vi "dds_rom_mixer_filter_spi.vi"() -> ()   [LabVIEW 2018]
uses:
  <vilib>/Analysis/NI_AALBase.lvlib
panel:
  out "IVAL":i16
  in  "Load":bool
  in  "ADC Offset":u16
  in  "PID":cluster{"S":i16, "O":i16, "P":i16, "I":i8}
  in  "Port":refnum<visa-resource-name>="COM3"
  in  "Init":bool
  in  "DDS":T1(array[cluster])=[{"Frequency"=0, "Attenuation"=0, "Phase"=0.0}, {"Frequency"=0, "Attenuation"=0, "Phase"=0.0}] {"Phase" min=0.0 max=2.0 format="%.3f"; "Attenuation" max=15}
  in  "Y":u16(ring)=4 items=["DDS0", "DDS1", "ROM", "MIXER", "FILTER", "ADC0", "ADC1", "ADC2", "ADC12", "PID"]
  in  "X":u16(ring) items=["DDS0", "DDS1", "ROM", "MIXER", "FILTER", "ADC0", "ADC1", "ADC2", "ADC12", "PID"]
  in  "t":u16(ring) items=["DDS", "ROM", "MIXER", "FILTER", "DAC", "ADC", "PID"]
  in  "State":u16(ring) items=["IDLE", "TEST", "DDS_DAC", "DDS_DAC_FILTER", "ADC", "DDS_DAC_ADC", "DDS_DAC_ADC_MIXER_FILTER", "DDS_DAC_ADC_MIXER_FILTER_PID"]
  in  "Filter Param":u16=9 max=15
  in  "stop":bool
  out "Waveform Graph":i16[][](graph)
  out "XY Graph":cluster{i16[], i16[]}(graph)
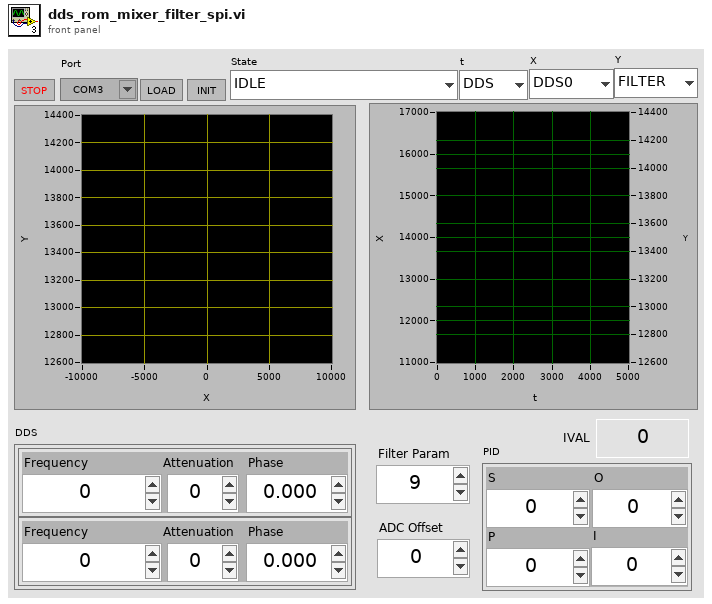
[diagram p1: front panel]
types:
  T1 = cluster{"Frequency":u16, "Attenuation":u16, "Phase":dbl}[]
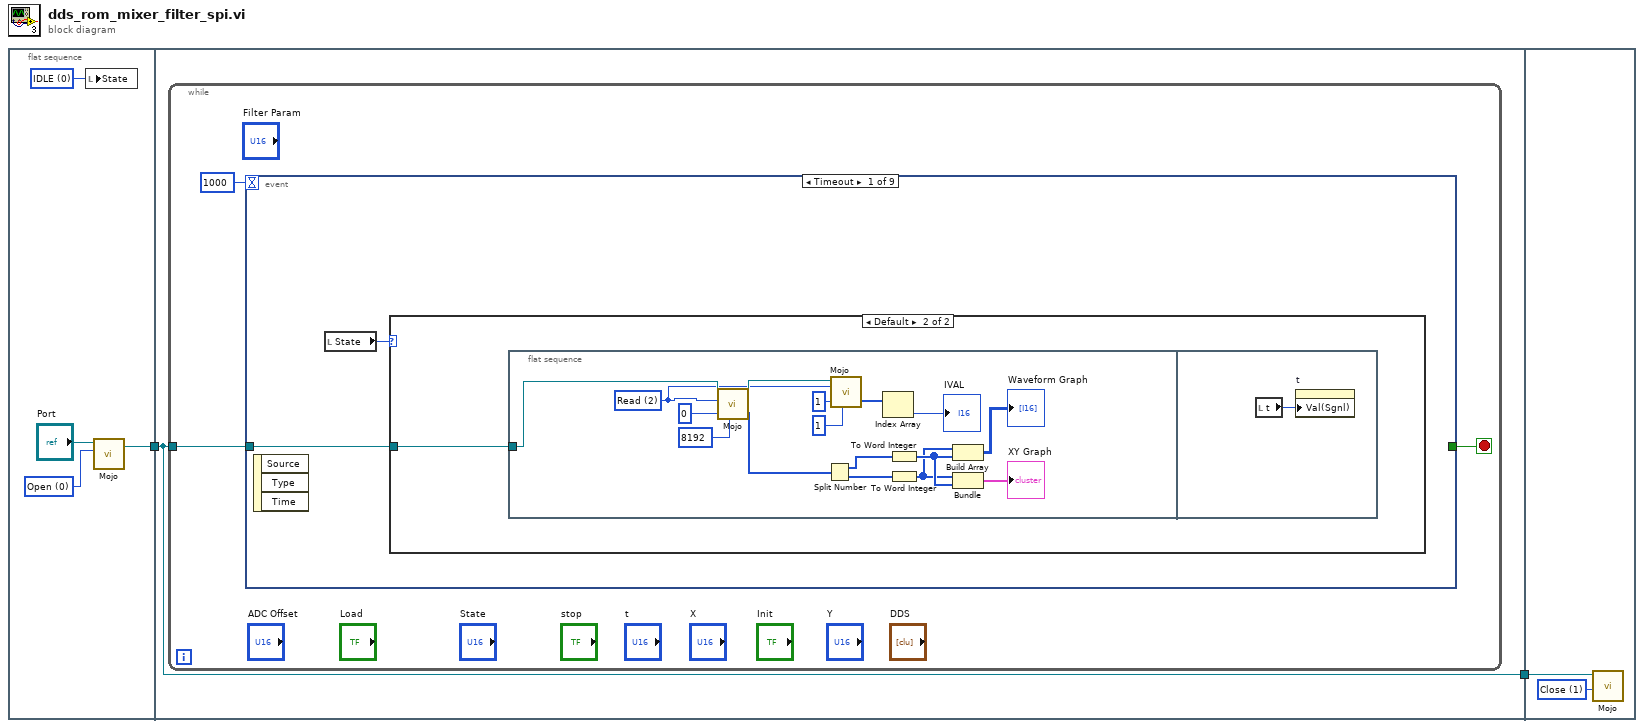
[diagram p0: block diagram]
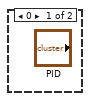
[diagram p2: hidden frame]
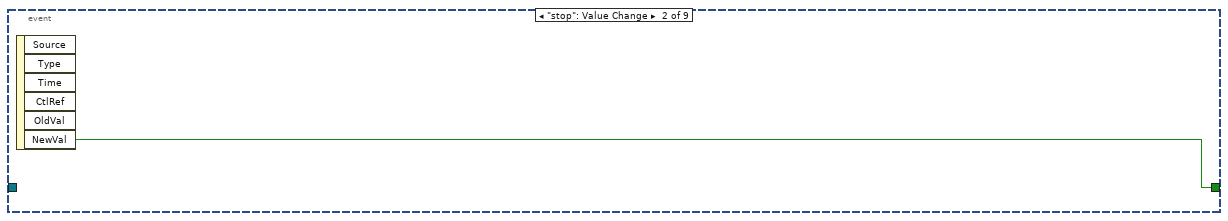
[diagram p3: hidden frame]
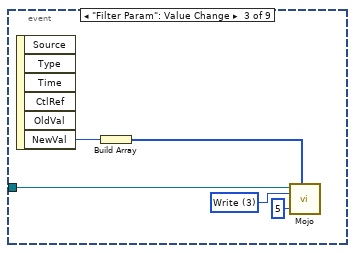
[diagram p4: hidden frame]
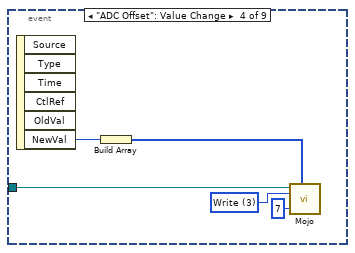
[diagram p5: hidden frame]
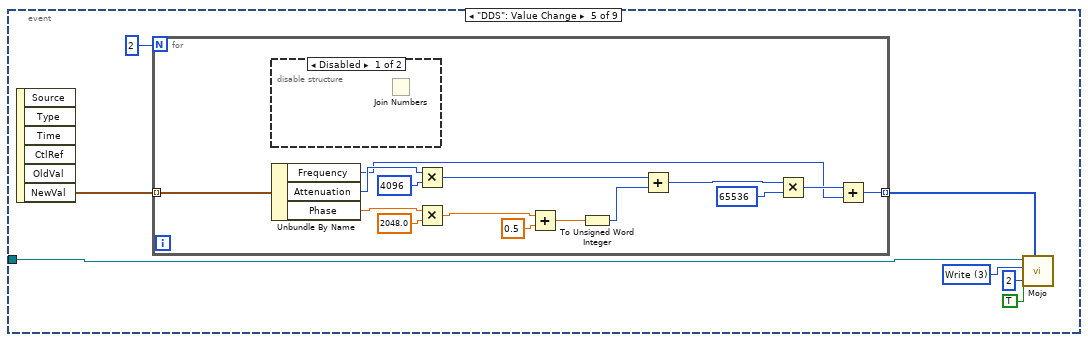
[diagram p6: hidden frame]
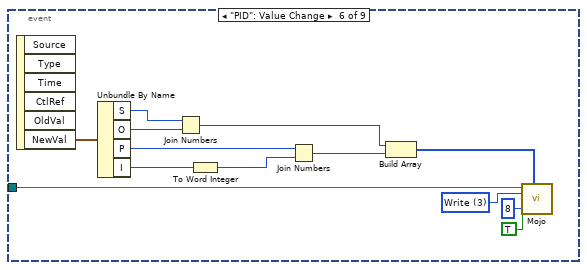
[diagram p8: hidden frame]
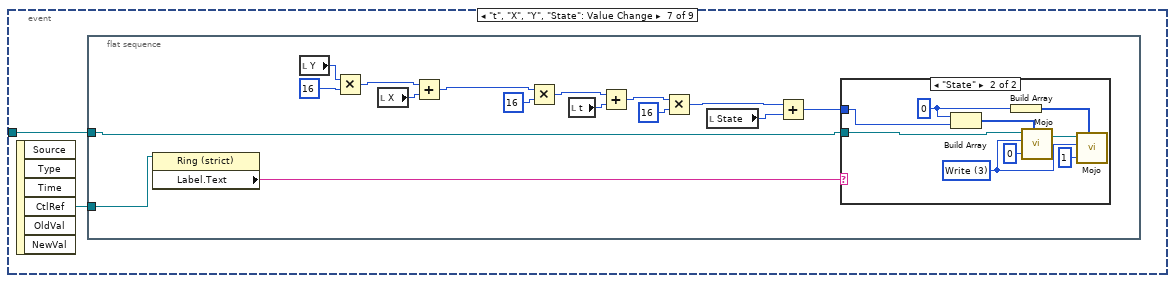
[diagram p9: hidden frame]
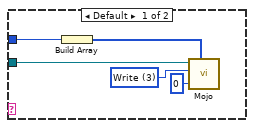
[diagram p10: hidden frame]
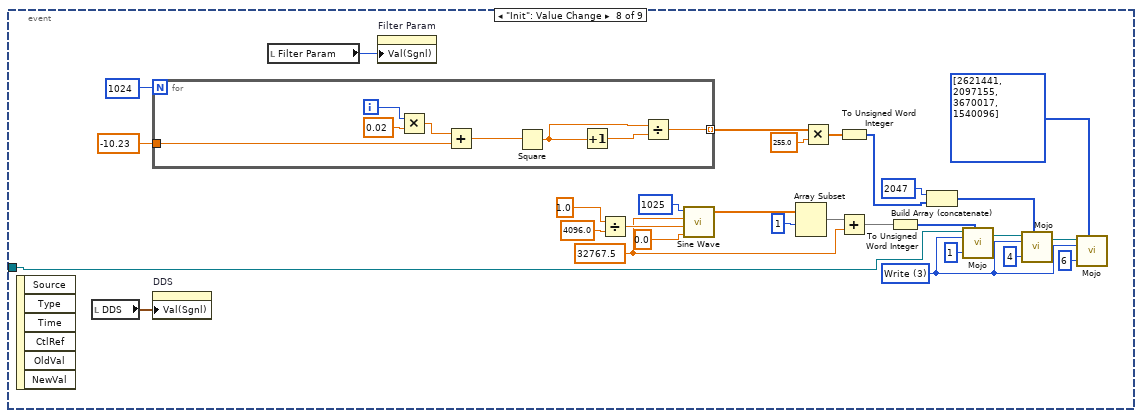
[diagram p11: hidden frame]
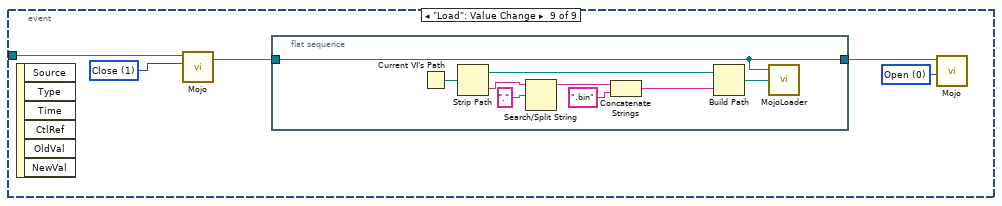
[diagram p12: hidden frame]
diagram:
  n1 = flat-sequence {
    tunnel: [w4] -> w2
    tunnel: w2 -> [w7]
    tunnel: [w7] -> w1
    tunnel: w1 -> [w160]
    frame #0 {
      w3 = u16 0 items=["IDLE", "TEST", "DDS_DAC", "DDS_DAC_FILTER", "ADC", "DDS_DAC_ADC", "DDS_DAC_ADC_MIXER_FILTER", "DDS_DAC_ADC_MIXER_FILTER_PID"] ("State")
      w5 = u8 0 items=["Open", "Close", "Read", "Write"] ("Mode")
      n2 = local write "State"(w3) -> ()
      n3 = call "Mojo.vi"("Mode"=w5, "Port In"="Port") -> ("Port Out"=w4:refnum<visa-resource-name>)  [unwired: 4 in, 1 out]
    }
    frame #1 {
      n4 = while {
        tunnel: w7 -> [w8]
        stop <- w10 stop-if-true
        n5 = event shown="[0] Timeout" {
          selector: _ -> [_ _ _ _ _ _ _ _ _]
          dyn-events: _ -> [_ _ _ _ _ _ _ _ _]
          timeout: 1000 -> [_ _ _ _ _ _ _ _ _]
          tunnel: [_ w31 _ _ _ _ _ _ _] -> w10
          tunnel: w8 -> [w12 _ w32 w37 w42 w72 w77 w115 w148]
          event Timeout {
            n6 = event-data() -> ()  [unwired: 1 in, 3 out]
            n7 = local read "State"() -> (w11:u16)
            n8 = case shown="Default" w11 {
              tunnel: w12 -> [_ w13]
              frame 0 {
              }
              frame Default {
                n9 = flat-sequence {
                  tunnel: w13 -> [w26]
                  frame #0 {
                    w18 = u8 2 items=["Open", "Close", "Read", "Write"] ("Mode")
                    n10 = call "Mojo.vi"("Length"=i16 8192, "Address"=u32 0, "Mode"=w18, "Port In"=w26) -> ("Data Out"=w20:i32[], "Port Out"=w19:refnum<visa-resource-name>)  [unwired: 2 in]
                    n11 = Split Number(x=w20) -> (hi(x)=w24:u16[], lo(x)=w22:u16[])
                    n12 = call "Mojo.vi"("Length"=i16 1, "Address"=u32 1, "Mode"=w18, "Port In"=w19) -> ("Data Out"=w15:i32[])  [unwired: 2 in, 1 out]
                    n13 = Index Array(array=w15) -> (element=→"IVAL":i32)  [unwired: 1 in]
                    n14 = To Word Integer(number=w24) -> (16bit integer=w23:i16[])
                    n15 = To Word Integer(number=w22) -> (16bit integer=w21:i16[])
                    n16 = Build Array(w21, w23) -> (→"Waveform Graph":i16[][])
                    n17 = Bundle(w21, w23) -> (→"XY Graph":cluster{i16[], i16[]})  [unwired: 1 in]
                  }
                  frame #1 {
                    n18 = local read "t"() -> (w30:u16)
                    n19 = property on="t" class="Ring (strict)"("Val(Sgnl)"=w30) -> ()  [unwired: 2 in, 2 out]
                  }
                }
              }
            }
          }
          event "stop": Value Change {
            n20 = event-data() -> ("NewVal"=w31:bool)  [unwired: 1 in, 5 out]
          }
          event "Filter Param": Value Change {
            w36 = u8 3 items=["Open", "Close", "Read", "Write"] ("Mode")
            n21 = event-data() -> ("NewVal"=w34:u16)  [unwired: 1 in, 5 out]
            n22 = Build Array(w34) -> (w33:u16[])
            n23 = call "Mojo.vi"("Data In"=w33, "Address"=u32 5, "Mode"=w36, "Port In"=w32) -> ()  [unwired: 2 in, 2 out]
          }
          event "ADC Offset": Value Change {
            w41 = u8 3 items=["Open", "Close", "Read", "Write"] ("Mode")
            n24 = event-data() -> ("NewVal"=w39:u16)  [unwired: 1 in, 5 out]
            n25 = Build Array(w39) -> (w38:u16[])
            n26 = call "Mojo.vi"("Data In"=w38, "Address"=u32 7, "Mode"=w41, "Port In"=w37) -> ()  [unwired: 2 in, 2 out]
          }
          event "DDS": Value Change {
            w46 = u8 3 items=["Open", "Close", "Read", "Write"] ("Mode")
            n27 = event-data() -> ("NewVal"=w47:T1)  [unwired: 1 in, 5 out]
            n28 = for {
              N: 2 -> [_]
              tunnel: w47 -> [w63] mode=indexing
              tunnel: [w54] -> w43 mode=indexing
              n29 = disable-structure shown="Disabled" {
                frame Disabled {
                  n30 = Join Numbers() -> ()  [unwired: 2 in, 1 out]
                }
                frame Enabled {
                }
              }
              n31 = Unbundle By Name(w63) -> ("Frequency"=w55:u16, "Attenuation"=w61:u16, "Phase"=w59:dbl)
              n32 = Multiply(x=w61, y=u32 4096) -> (x*y=w60:u32)
              n33 = Multiply(x=w59, y=2048.0) -> (x*y=w52:dbl)
              n34 = Add(x=w52, y=0.5) -> (x+y=w50:dbl)
              n35 = To Unsigned Word Integer(number=w50) -> (unsigned 16bit integer=w49:u16)
              n36 = Add(x=w60, y=w49) -> (x+y=w58:u32)
              n37 = Multiply(x=w58, y=u32 65536) -> (x*y=w56:u32)
              n38 = Add(x=w56, y=w55) -> (x+y=w54:u32)
            }
            n39 = call "Mojo.vi"("Data In"=w43, "Increment"=TRUE, "Address"=u32 2, "Mode"=w46, "Port In"=w42) -> ()  [unwired: 1 in, 2 out]
          }
          event "PID": Value Change {
            w75 = u8 3 items=["Open", "Close", "Read", "Write"] ("Mode")
            n40 = event-data() -> ("NewVal"=w76:cluster{"S":i16, "O":i16, "P":i16, "I":i8})  [unwired: 1 in, 5 out]
            n41 = Unbundle By Name(w76) -> ("S"=w70:i16, "O"=w71:i16, "P"=w69:i16, "I"=w65:i8)
            n42 = Join Numbers(hi=w70, lo=w71) -> ((hi.lo)=w68:u32)
            n43 = To Word Integer(number=w65) -> (16bit integer=w64:i16)
            n44 = Join Numbers(hi=w69, lo=w64) -> ((hi.lo)=w67:u32)
            n45 = Build Array(w68, w67) -> (w66:u32[])
            n46 = call "Mojo.vi"("Data In"=w66, "Increment"=TRUE, "Address"=u32 8, "Mode"=w75, "Port In"=w72) -> ()  [unwired: 1 in, 2 out]
          }
          event "t", "X", "Y", "State": Value Change {
            n47 = event-data() -> ("CtlRef"=w78:refnum<vi>)  [unwired: 1 in, 5 out]
            n48 = flat-sequence {
              tunnel: w78 -> [w82]
              tunnel: w77 -> [w79]
              frame #0 {
                n49 = property class="Ring (strict)"(reference=w82) -> ("Label.Text"=w81:string)  [unwired: 1 in, 2 out]
                n50 = local read "Y"() -> (w92:u16)
                n51 = Multiply(x=w92, y=u32 16) -> (x*y=w93:u32)
                n52 = local read "X"() -> (w91:u16)
                n53 = Add(x=w93, y=w91) -> (x+y=w89:u32)
                n54 = Multiply(x=w89, y=u32 16) -> (x*y=w88:u32)
                n55 = local read "t"() -> (w87:u16)
                n56 = Add(x=w88, y=w87) -> (x+y=w85:u32)
                n57 = Multiply(x=w85, y=u32 16) -> (x*y=w84:u32)
                n58 = local read "State"() -> (w83:u16)
                n59 = Add(x=w84, y=w83) -> (x+y=w80:u32)
                n60 = case shown="\"State\"" w81 {
                  tunnel: w80 -> [w98 w107]
                  tunnel: w79 -> [w95 w100]
                  frame Default {
                    w96 = u8 3 items=["Open", "Close", "Read", "Write"] ("Mode")
                    n61 = Build Array(w98) -> (w99:u32[])
                    n62 = call "Mojo.vi"("Data In"=w99, "Address"=u32 0, "Mode"=w96, "Port In"=w95) -> ()  [unwired: 2 in, 2 out]
                  }
                  frame "State" {
                    w102 = u32 0 ("element")
                    w104 = u8 3 items=["Open", "Close", "Read", "Write"] ("Mode")
                    n63 = Build Array(w102, w107) -> (w106:u32[])
                    n64 = Build Array(w102) -> (w101:u32[])
                    n65 = call "Mojo.vi"("Data In"=w106, "Address"=u32 0, "Mode"=w104, "Port In"=w100) -> ("Port Out"=w105:refnum<visa-resource-name>)  [unwired: 2 in, 1 out]
                    n66 = call "Mojo.vi"("Data In"=w101, "Address"=u32 1, "Mode"=w104, "Port In"=w105) -> ()  [unwired: 2 in, 2 out]
                  }
                }
              }
            }
          }
          event "Init": Value Change {
            w109 = u8 3 items=["Open", "Close", "Read", "Write"] ("Mode")
            w129 = 32767.5 ("amplitude")
            n67 = event-data() -> ()  [unwired: 1 in, 6 out]
            n68 = local read "DDS"() -> (w113:T1)
            n69 = for {
              N: 1024 -> [_]
              tunnel: -10.23 ("amplitude") -> [w142]
              tunnel: [w138] -> w123 mode=indexing
              i -> [w145]
              n70 = Multiply(x=w145, y=0.02) -> (x*y=w143:dbl)
              n71 = Add(x=w143, y=w142) -> (x+y=w141:dbl)
              n72 = Square(x=w141) -> (x^2=w139:dbl)
              n73 = Increment(x=w139) -> (x+1=w140:dbl)
              n74 = Divide(x=w139, y=w140) -> (x/y=w138:dbl)
            }
            n75 = property on="DDS" class="Arr (strict)"("Val(Sgnl)"=w113) -> ()  [unwired: 2 in, 2 out]
            n76 = local read "Filter Param"() -> (w114:u16)
            n77 = property on="Filter Param" class="DigNum (strict)"("Val(Sgnl)"=w114) -> ()  [unwired: 2 in, 2 out]
            n78 = Divide(x=1.0 ("frequency"), y=4096.0) -> (x/y=w135:dbl)
            n79 = call <vilib>:"Sine Wave.vi"("samples"=1025, "amplitude"=w129, "frequency"=w135, "phase in"=0.0 ("phase")) -> ("sine wave"=w132:dbl[])  [unwired: 1 in, 2 out]
            n80 = Array Subset(array=w132, index=1) -> (w130:dbl[])  [unwired: 1 in]
            n81 = Multiply(x=w123, y=255.0 ("amplitude")) -> (x*y=w121:dbl[])
            n82 = To Unsigned Word Integer(number=w121) -> (unsigned 16bit integer=w118:u16[])
            n83 = Add(x=w130, y=w129) -> (x+y=w128:dbl[])
            n84 = To Unsigned Word Integer(number=w128) -> (unsigned 16bit integer=w127:u16[])
            n85 = Build Array (concatenate)(2047, w118) -> (w117:i32[])
            n86 = call "Mojo.vi"("Data In"=w127, "Address"=u32 1, "Mode"=w109, "Port In"=w115) -> ("Port Out"=w120:refnum<visa-resource-name>)  [unwired: 2 in, 1 out]
            n87 = call "Mojo.vi"("Data In"=w117, "Address"=u32 4, "Mode"=w109, "Port In"=w120) -> ("Port Out"=w111:refnum<visa-resource-name>)  [unwired: 2 in, 1 out]
            n88 = call "Mojo.vi"("Data In"=i32[] [2621441, 2097155, 3670017, 1540096] ("appended array"), "Address"=u32 6, "Mode"=w109, "Port In"=w111) -> ()  [unwired: 2 in, 2 out]
          }
          event "Load": Value Change {
            w149 = u8 1 items=["Open", "Close", "Read", "Write"] ("Mode")
            w150 = u8 0 items=["Open", "Close", "Read", "Write"] ("Mode")
            n89 = event-data() -> ()  [unwired: 1 in, 6 out]
            n90 = call "Mojo.vi"("Mode"=w149, "Port In"=w148) -> ("Port Out"=w147:refnum<visa-resource-name>)  [unwired: 4 in, 1 out]
            n91 = flat-sequence {
              tunnel: w147 -> [w159]
              tunnel: [w159] -> w146
              frame #0 {
                n92 = Current VI's Path() -> (path=w156:path)
                n93 = Strip Path(path=w156) -> (stripped path=w152:path, name=w158:string)
                n94 = Search/Split String(string=w158, search string/char (-)=".") -> (substring before match=w155:string)  [unwired: 1 in, 2 out]
                n95 = Concatenate Strings(w155, ".bin" ("string")) -> (w153:string)
                n96 = Build Path(base path=w152, name or relative path=w153) -> (appended path=w151:path)
                n97 = call "MojoLoader.vi"("Path"=w151, "Port"=w159) -> ()  [unwired: 1 in]
              }
            }
            n98 = call "Mojo.vi"("Mode"=w150, "Port In"=w146) -> ()  [unwired: 4 in, 2 out]
          }
        }
      }
    }
    frame #2 {
      w161 = u8 1 items=["Open", "Close", "Read", "Write"] ("Mode")
      n99 = call "Mojo.vi"("Mode"=w161, "Port In"=w160) -> ()  [unwired: 4 in, 2 out]
    }
  }
